vi "Start Test Time.vi"() -> (1 "Test Start Time":string)   [LabVIEW 2016]
panel:
  out "时间字符串":string
  out "日期字符串":string
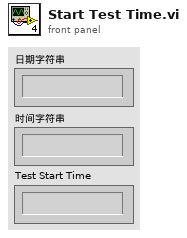
[diagram p1: front panel]
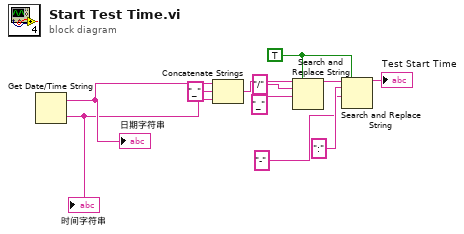
[diagram p0: block diagram]
diagram:
  w6 = TRUE ("替换全部？(F)")
  n1 = Get Date/Time String() -> (date string=w11:string, time string=w9:string)  [unwired: 3 in]
  "日期字符串" <- w11
  "时间字符串" <- w9
  n2 = Concatenate Strings(w11, "_" ("字符串"), w9) -> (w10:string)
  n3 = Search and Replace String(replace all?=w6, input string=w10, search string="/" ("搜索字符串"), replace string="_" ("替换字符串(\"\")")) -> (result string=w5:string)  [unwired: 4 in, 3 out]
  n4 = Search and Replace String(replace all?=w6, input string=w5, search string=":" ("搜索字符串"), replace string="-" ("替换字符串(\"\")")) -> (result string=→"Test Start Time":string)  [unwired: 4 in, 3 out]
